vi "Dashboard Main.vi"() -> ()   [LabVIEW 2014]
uses:
  <vilib>/Rock Robotics/WPI/DriverStation/WPI_DriverStationRobotMode2.ctl
  <vilib>/event_ctls.llb/eventvkey.ctl
  <vilib>/Rock Robotics/WPI/Dashboard/WPI_DashboardLogging Global.vi
  <vilib>/Rock Robotics/Network Tables/SD Write Number.vi
  <vilib>/Rock Robotics/Network Tables/NT Read Numeric Array.vi
  <vilib>/Rock Robotics/Network Tables/SD Read Number.vi
  <vilib>/Rock Robotics/Network Tables/SD Write Boolean.vi
  <vilib>/Utility/config.llb/Write Key (String).vi
  <vilib>/Utility/config.llb/Write Key (I32).vi
  <vilib>/Utility/config.llb/Read Key (I32).vi
  <vilib>/Utility/config.llb/Read Key (Double).vi
  <vilib>/Utility/config.llb/Write Key (Double).vi
  <vilib>/Utility/config.llb/NI_LVConfig.lvlib
panel:
  in  "TCP":refnum<k5>
  out "Camera IP":string
  out "Image Message":string="Timeout in Camera Communications"
  in  "Dashboard Tab":T1(tab)
  in  "Straight Forward":bool
  in  "Camera Settings":T2={"Frame Rate"=30, "Compression"=30, "Size"=1} {"Frame Rate" scale=1.0..30.0; "Size" items=["640x480", "320x240", "160x120"]}
  out "MotorChart R":cluster{"Numeric":dbl, "Numeric":dbl}(graph)
  out "MotorChart L":T3(graph)
  out "MotorSliders R":cluster{"MotorSlide1":dbl, "MotorSlide2":dbl} {"MotorSlide2" scale=-1.0..1.0 scale format="%#_2e"; "MotorSlide1" scale=-1.0..1.0 scale format="%#_2e"}
  out "MotorSliders L":T4 {"MotorSlide4 2" scale=0.0..14.0 scale format="%#_2e"; "MotorSlide2" scale=-1.0..1.0 scale format="%#_2e"; "MotorSlide1" scale=-1.0..1.0 scale format="%#_2e"}
  out "Yaw":dbl(knob) scale=180.0..-180.0
  out "JS1 Z":dbl(slide) scale=-1.0..1.0 scale format="%#_2e"
  out "JS1 Graph":cluster{"X":dbl, "Y":dbl}[](graph)
  out "JS1 Buttons":T5
  out "JS2 Z":dbl(slide) scale=-1.0..1.0 scale format="%#_2e"
  out "JS2 Graph":cluster{"X":dbl, "Y":dbl}[](graph)
  out "JS2 Buttons":T5
  out "Mode":T6(ring)=enum."Auto Disabled"
  in  "DB Camera Config":bool
  out "fps":dbl format="%#.1g"
  out "Mbps":dbl format="%#.1g"
  out "Mbps 2":bool
  in  "Use This Auto":enum16{"Grab", "Knock", "Drive", "Test"}(ring)
  in  "Load":bool
  in  "Save":bool
  in  "Actions":T7(array[ring])
  in  "Bin Z":dbl
  in  "Gap Y":dbl
  in  "Auto Zone Y":dbl
  in  "Bin 4 Coordinates":dbl[](array[numeric])=[117.35, 90.0]
  in  "Bin 3 Coordinates":dbl[](array[numeric])=[48.65, 90.0]
  in  "Bin 2 Coordinates":dbl[](array[numeric])=[-48.65, 90.0]
  in  "Bin 1 Coordinates":dbl[](array[numeric])=[-117.35, 90.0]
  in  "Middle 2 Bins":enum16{"Strafe By", "Go Into Gap"}(ring)
  in  "Auto Zone":enum16{"0", "1", "2", "3", "4"}(ring)
  in  "Start Position":T8(ring)
  in  "In. to go forward":dbl format="%#_13g"
  out "CAN Device Errors":dbl[](array[numeric])
  out "Waveform Chart":T9(graph)
  in  "Test Slider":dbl(slide) scale=0.0..100.0 scale format="%#_3g"
  in  "On/Off":bool caption="Solenoid"
  in  "Test Name":u16(ring) items=["Select the test to run...", "Example Test", "-------------------------------", "List of tests is built in robot code.", "Replace with your own automated tests."]
  in  "Test Tree":string(tree)
  in  "Motor":cluster{"Value":dbl, "Enable":bool} {"Value" scale=-1.0..1.0 scale format="%#_3g"}
  out "Progress":T10 {"Test Progress" scale=0.0..100.0}
  in  "Rev/Fwd":cluster{"Forward":bool, "Reverse":bool}
  in  "Test Ring":u16(ring) items=["Monochrome", "Color"]
  in  "Vision":u16(ring) items=["Camera Off", "USB Camera SW", "USB Camera HW", "IP Camera"]
  in  "Rec Mode":enum32{"Stop", "Record", "Playback"}(radio)
  in  "Listbox":i32(listbox)
  out "Tree":string(tree)
  out "Camera Image":T11(plugin-control)
  out "Boolean":bool
  # "Left"
  # "Front"
  # "Right"
  # "Battery"
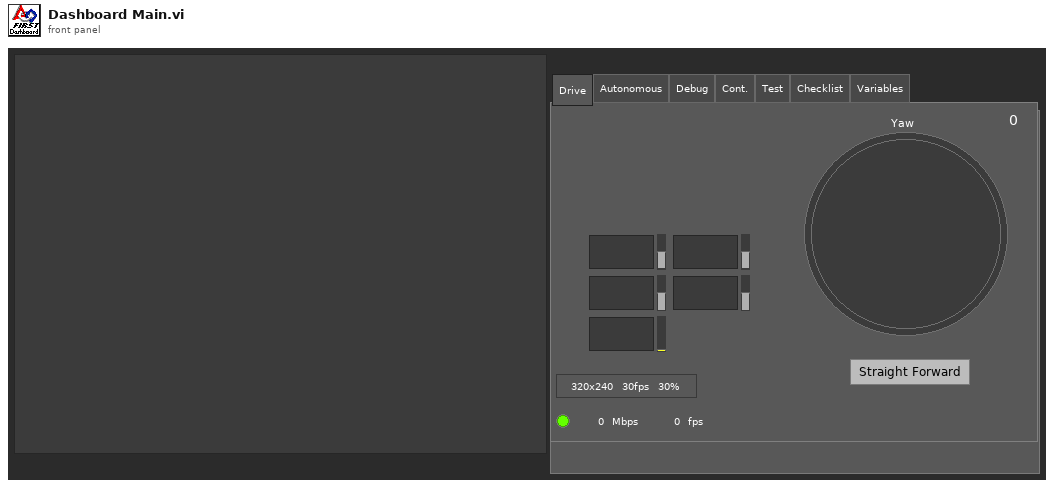
[diagram p1: front panel]
types:
  T1 = enum32{"Drive", "Autonomous", "Debug", "Cont.", "Test", "Checklist", "Variables"}
  T2 = cluster{"Frame Rate":i32, "Compression":i32, "Size":u16}
  T3 = cluster{"Numeric":dbl, "Numeric":dbl, "Battery V":dbl}
  T4 = cluster{"MotorSlide1":dbl, "MotorSlide2":dbl, "MotorSlide4 2":dbl}
  T5 = cluster{bool, bool, bool, bool, bool, bool, bool, bool, bool, bool, bool, bool}
  T6 = enum8{"Tele-Op Disabled", "Tele-Op Enabled", "Auto Disabled", "Auto Enabled", "Test Disabled", "Test Enabled", "Disconnected", "No Code", "E-Stop"}
  T7 = enum16{"Go To Auto Zone", "Grab Bin 1", "Grab Bin 2", "Grab Bin 3", "Grab Bin 4"}[]
  T8 = enum16{"Bin 1", "Bin 2", "Middle", "Bin 3", "Bin 4"}
  T9 = cluster{"Numeric Array[0]":dbl, "Numeric Array[1]":dbl, "Numeric Array[2]":dbl, "Numeric Array[3]":dbl, "Numeric Array[4]":dbl, "Numeric Array[5]":dbl, "Numeric Array[6]":dbl, "Numeric Array[7]":dbl, "Numeric Array[8]":dbl, "Numeric Array[9]":dbl}
  T10 = cluster{"Test Progress":u8, "Test Progress Text":string}
  T11 = typedef "IMAQ Image.ctl" = refnum<image>
  T12 = enum32{"Drive", "Basic", "Custom", "Test", "Checklist", "Variables"}
  T13 = typedef "Image Type" = u32
  T14 = typedef "NI_LVConfig.lvlib/Config Data RefNum.ctl" = refnum<k1>
  T15 = typedef "WPI_DriverStationRobotMode2.ctl" = enum16{"Autonomous Disabled", "Autonomous Enabled", "Teleop Disabled", "Teleop Enabled", "Disconnected", "Finish", "Test Disabled", "Test Enabled", "Emergency Stopped"}
  T16 = enum16{"Go To Auto Zone", "Grab Bin 1", "Grab Bin 2", "Grab Bin 3", "Grab Bin 4"}
  T17 = cluster{"Camera Image":refnum<vi>, "Dashboard Tab":refnum<vi>, "Boolean":refnum<vi>, "Vision":refnum<vi>, "Rec Mode":refnum<vi>, "Test Slider":refnum<vi>, "On/Off ":refnum<vi>, "Test Ring":refnum<vi>, "Rev/Fwd":refnum<vi>, "Test Name":refnum<vi>, "Motor":refnum<vi>, "Progress":refnum<vi>, "CheckList":refnum<vi>, "Tree":refnum<vi>, "Test Tree":refnum<vi>}
  T18 = cluster{"Error Strings":string, "Disable Counts":cluster{u16, u16}, "Rail Faults":cluster{u16, u16, u16}, "Robot IP":string, "DB Mode":u8, "Event Info":cluster{"Name":string, "Type":u8, "Number":u16, "Replay":u8}, "Camera Addr":string}
  T19 = cluster{"Storage":cluster{"Disk Free":u64, "RAM Block":u32, "RAM free":u32}, "CPU Utilization":cluster{"CPU % ISR":sgl, "CPU % Time Crit":sgl, "CPU % Timed Str":sgl, "CPU % High":sgl, "CPU % Above":sgl, "CPU % Normal":sgl, "CPU % Low":sgl}, "CAN":cluster{"% Bus Utilization":sgl, "Bus Off Cnt":u32, "TX_FIFO Full Cnt":u32, "Receive Error Cnt":u8, "Transmit Error Cnt":u8}, "HID":cluster{"HID Outputs":u32, "Rumble Low":u16, "Rumble High":u16}[]}
  T20 = cluster{"Status bits":cluster{"Test Mode":bool, "Autonomous":bool, "Enabled":bool, "Code Start":bool, "Brownout":bool, "Reserved 2":bool, "Reserved 3":bool, "E-Stop":bool}, "Code Trace":cluster{"Disabled":bool, "TeleOp":bool, "Auto":bool, "Test":bool}, "Controller Type":enum16{"unknown", "cRIO", "roboRio"}, "Code?":enum16{"unknown", "noCode", "code"}, "Battery V":dbl}
  T21 = cluster{"Control Bits":cluster{"TestMode":bool, "Autonomous":bool, "Enabled":bool, "FMS Present":bool, bool, bool, bool, "E-Stop":bool}, "Team Station ":u8, "Countdown":sgl, "Joystick Values":cluster{"Axes":dbl[], "Buttons":bool[], "POVs":i16[]}[]}
  T22 = cluster{"Axes":dbl[], "Buttons":bool[], "POVs":i16[]}[]
  T23 = cluster{"Axes":dbl[], "Buttons":bool[], "POVs":i16[]}
  T24 = cluster{"Buttons[0]":bool, "Buttons[1]":bool, "Buttons[2]":bool, "Buttons[3]":bool, "Buttons[4]":bool, "Buttons[5]":bool, "Buttons[6]":bool, "Buttons[7]":bool, "Buttons[8]":bool, "Buttons[9]":bool, "Buttons[10]":bool, "Buttons[11]":bool}
  T25 = cluster{"Operation":enum16{"Update", "Clear"}, "Color Box":u32}[]
  T26 = typedef "eventvkey.ctl" = enum16{"ASCII", "Enter", "Return", "Shift", "Ctrl", "Alt", "Cmd", "Opt", "Caps", "NumLock", "Clear", "Break", "Up", "Down", "Left", "Right", "Insert", "Delete", "Home", "End", "PageUp", "PageDown", "Escape", "Help", "Pause", "ScrollLock", "F1", "F2", "F3", "F4", "F5", "F6", "F7", "F8", "F9", "F10", "F11", "F12", "F13", "F14", "F15", "F16", "F17", "F18", "F19", "F20", "F21", "F22", "F23", "F24", "Play", "VolumeUp", "VolumeDown", "Mute", "Two Byte Char"}
  T27 = cluster{"Image Size":bool, "Image Type":bool, "Pixel Value":bool, "ROI Information":bool, "Zoom Factor":bool}
  T28 = enum8{"Enabled", "Disabled", "Disabled and Grayed Out"}
  T29 = cluster{"Operation":enum16{"Update", "Clear"}, "Color Box":u32}
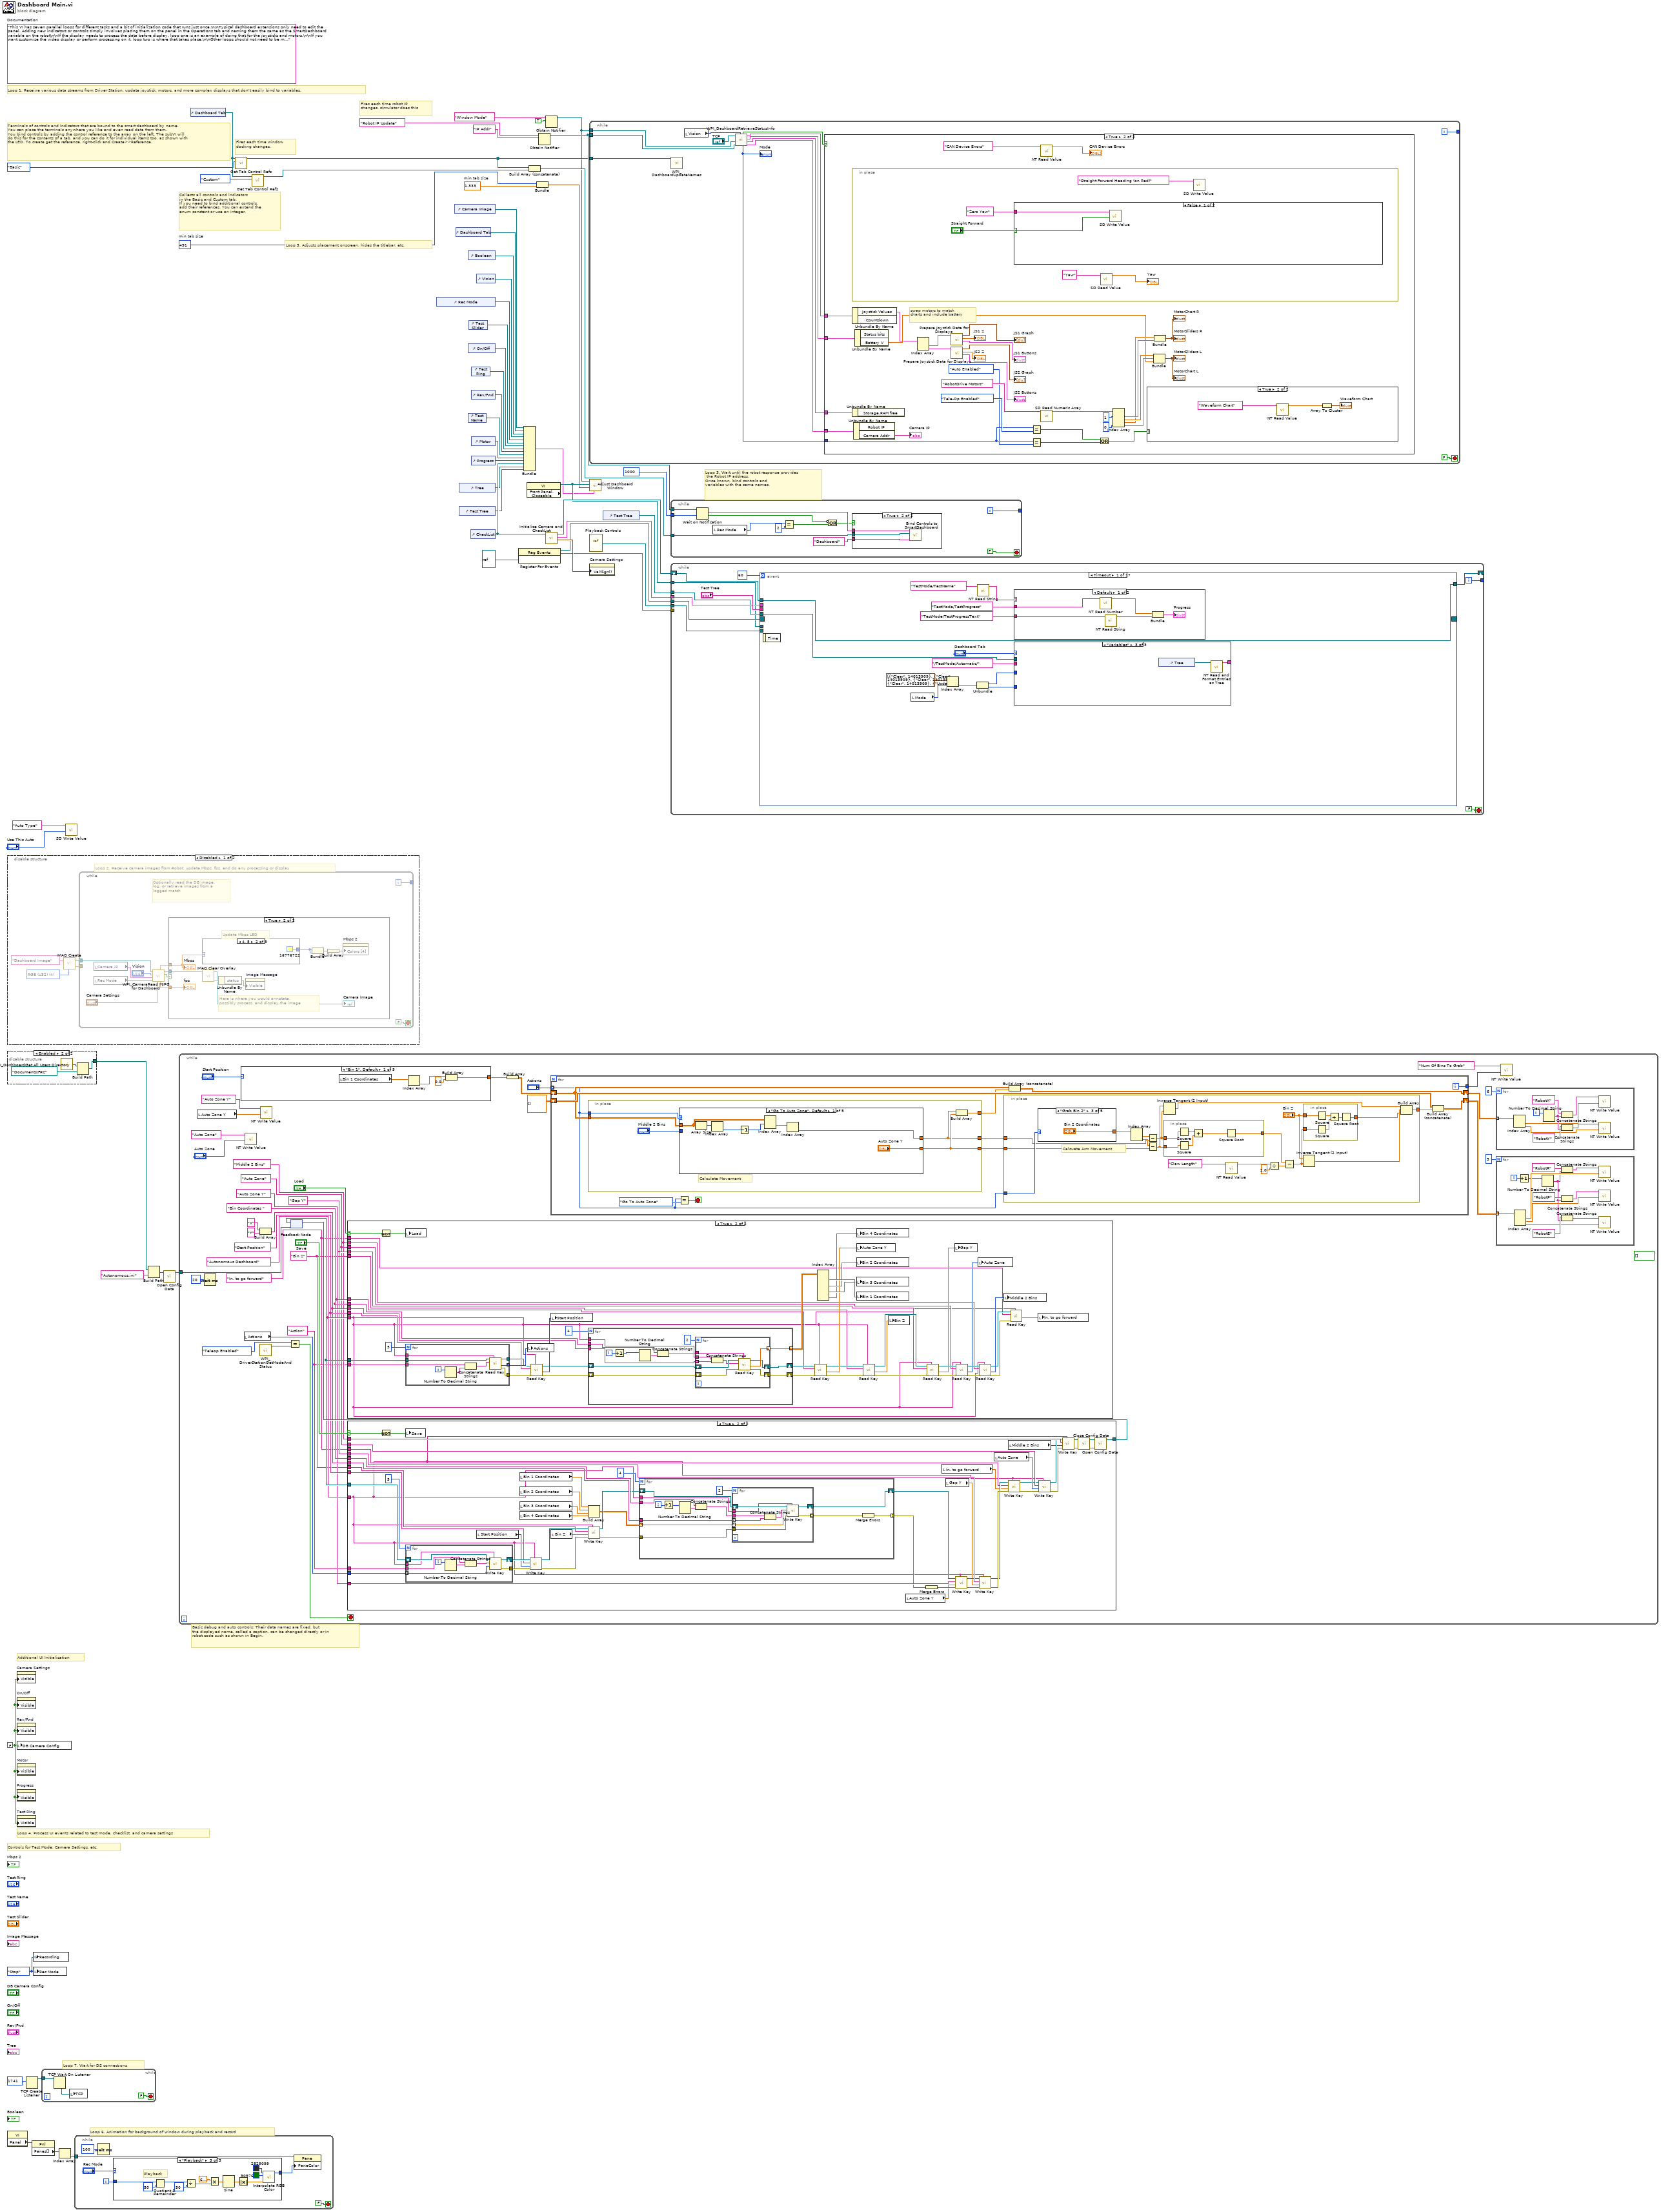
[diagram p0: block diagram]
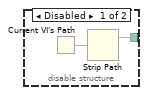
[diagram p2: hidden frame]
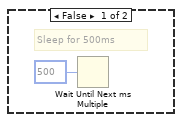
[diagram p3: hidden frame]
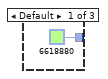
[diagram p4: hidden frame]
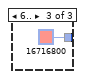
[diagram p5: hidden frame]
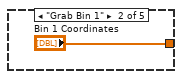
[diagram p10: hidden frame]
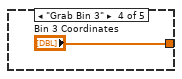
[diagram p11: hidden frame]
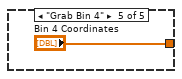
[diagram p12: hidden frame]
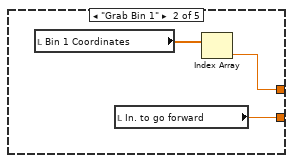
[diagram p13: hidden frame]
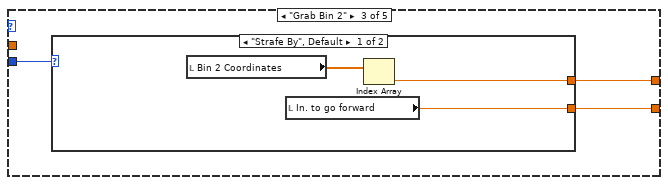
[diagram p14: hidden frame]
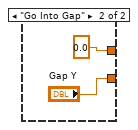
[diagram p15: hidden frame]
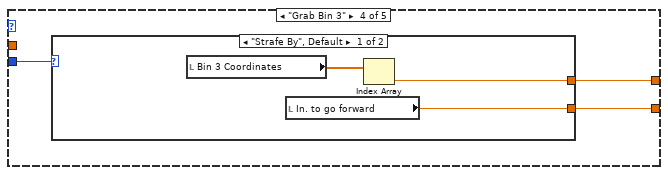
[diagram p16: hidden frame]
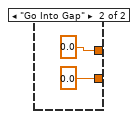
[diagram p17: hidden frame]
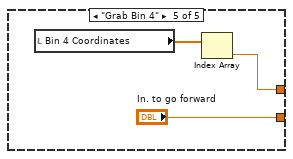
[diagram p18: hidden frame]
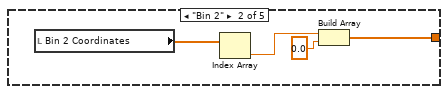
[diagram p19: hidden frame]
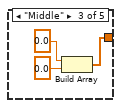
[diagram p20: hidden frame]
diagram:
  w30 = 491  # min tab size
  w29 = 1.333  # min tab size
  w38 = enum32{"Stop", "Record", "Playback"}."Stop" ("Rec Mode")
  w12 = FALSE ("Visible")
  (unwired) "This VI has seven parallel loops for different tasks and a bit of initialization code that runs just once.\n\nTypical dashboard extensions only need to edit the panel. Adding new indicators or controls simply involves placing them on the panel in the Operations tab and naming them the same as the SmartDashboard variable on the robot\n\nIf the display needs to process the data before display, loop one is an example of doing that for the joysticks and motors.\n\nIf you want customize the video display or perform processing on it, loop two is where that takes place.\n\nOther loops should not need to be modified. They are pretty standard, and document the task they perform."  # Documentation
  # "Loop 7. Wait for DS connections"
  # "Basic debug and auto controls: Their data names are fixed, but\nthe displayed name, called a caption, can be changed directly or in\nrobot code such as shown in Begin."
  # "Controls for Test Mode, Camera Settings, etc."
  # "Additional UI Initialization"
  # "Loop 6. Animation for background of window during playback and record"
  # "Fires each time robot IP\nchanges, simulator does this"
  # "Fires each time window\ndocking changes."
  # "Collects all controls and indicators\nin the Basic and Custom tab.\nIf you need to bind additional controls,\nadd their references. You can extend the\nenum constant or use an integer."
  # "Loop 4. Process UI events related to test mode, checklist, and camera settings"
  # "Terminals of controls and indicators that are bound to the smart dashboard by name.\nYou can place the terminals anywhere you like and even read data from them.\nYou bind controls by adding the control reference to the array on the left. The subVI will\ndo this for the contents of a tab, and you can do it for individual items too, as shown with\nthe LED. To create get the reference, right-click and Create>>Reference."
  # "Loop 3. Wait until the robot response provides\n the Robot IP address.\nOnce known, bind controls and\nvariables with the same names."
  # "Loop 5. Adjusts placement onscreen, hides the titlebar, etc."
  # "Loop 1. Receive various data streams from Driver Station, update joystick, motors, and more complex displays that don't easily bind to variables."
  n1 = disable-structure shown="Disabled" {
    frame Disabled {
      w58 = T13 4 items=["Grayscale (U8)", "Grayscale (I16)", "Grayscale (SGL)", "Complex (CSG)", "RGB (U32)", "HSL (U32)", "RGB (U64)"] ("Image Type")
      # "Loop 2. Receive camera images from Robot, update Mbps, fps, and do any processing or display"
      n2 = call "IMAQ Create"("Image Name"="Dashboard Image", "Image Type"=w58) -> ("New Image"=w56:T11, "error out"=w55:errorcluster)  [unwired: 2 in, 1 out]
      n3 = while {
        tunnel: w56 -> [w67]
        tunnel: w55 -> [_]
        tunnel: [w68] -> _
        i -> [w68]
        stop <- FALSE stop-if-true
        # "Optionally read the DB image,\nlog, or retrieve images from a\nlogged match"
        n4 = local read "Camera IP"() -> (w59:string)
        n5 = local read "Rec Mode"() -> (w61:enum32{"Stop", "Record", "Playback"})
        n6 = call <vilib>:"WPI_CameraRead MJPG for Dashboard.vi"("Camera Settings"="Camera Settings", "Rec Mode"=w61, "Camera IP"=w59, "Camera Mode"="Vision", "Refnum in"=w67) -> ("Active"=w65:bool, "Refnum out"=w66:T11, "FPS"=w64:dbl, "Bandwidth (Mbps)"=w63:dbl)  [unwired: 3 in]
        n7 = case shown="True" w65 {
          tunnel: w66 -> [_ w74]
          tunnel: w63 -> [_ w73]
          tunnel: w64 -> [_ w71]
          frame False {
            # "Sleep for 500ms"
            n8 = Wait Until Next ms Multiple(millisecond multiple=u32 500) -> ()  [unwired: 1 out]
          }
          frame True {
            # "Here is where you would annotate,\npossibly process, and display the image"
            # "Update Mbps LED"
            n9 = case shown="4, 5" w73 {
              tunnel: [u32 6618880 ("Color Box") u32 16776722 ("Color Box") u32 16716800 ("Color Box")] -> w75
              frame Default {
              }
              frame 4, 5 {
              }
              frame 6.. {
              }
            }
            n10 = call "IMAQ Clear Overlay"("Image"=w74) -> ("error out"=w78:errorcluster, "Image Out"=→"Camera Image":T11)  [unwired: 2 in, 7 out]
            n11 = Unbundle By Name(w78) -> ("status"=w79:bool)
            n12 = property on="Image Message" class="Str"("Visible"=w79) -> ()  [unwired: 2 in, 2 out]
            n13 = Bundle("Color Box"=w75, "Color Box"=w75) -> (w77:cluster{"Color Box":u32, "Color Box":u32})  [unwired: 1 out]
            n14 = Build Array(w77) -> (w76:cluster{"Color Box":u32, "Color Box":u32}[])
            n15 = property on="Mbps 2" class="Bool (strict)"("Colors [4]"=w76) -> ()  [unwired: 2 in, 2 out]
            "Mbps" <- w73
            "fps" <- w71
          }
        }
      }
    }
    frame Enabled {
    }
  }
  n16 = disable-structure shown="Enabled" {
    disable-tunnel: [w84 w87] -> w3
    frame Disabled {
      n17 = Current VI's Path() -> (path=w83:path)
      n18 = Strip Path(path=w83) -> (stripped path=w84:path)  [unwired: 1 out]
    }
    frame Enabled {
      n19 = call <vilib>:"WPI_DashboardGet All Users Directory.vi"() -> ("All User Path"=w85:path)
      n20 = Build Path(base path=w85, name or relative path=path "Documents/FRC" ("path")) -> (appended path=w87:path)
    }
  }
  n21 = property class="VI"() -> ("Panel"=w45:refnum<vi>)  [unwired: 2 in, 2 out]
  n22 = property on="Camera Settings" class="Clust (strict)"("Visible"=w12) -> ()  [unwired: 2 in, 2 out]
  n23 = property on="On/Off" class="Bool (strict)"("Visible"=w12) -> ()  [unwired: 2 in, 2 out]
  n24 = property on="Rev/Fwd" class="Clust (strict)"("Visible"=w12) -> ()  [unwired: 2 in, 2 out]
  n25 = local write "DB Camera Config"(w12) -> ()
  n26 = property on="Motor" class="Clust (strict)"("Visible"=w12) -> ()  [unwired: 2 in, 2 out]
  n27 = property on="Progress" class="Clust (strict)"("Visible"=w12) -> ()  [unwired: 2 in, 2 out]
  n28 = property on="Test Ring" class="Ring (strict)"("Visible"=w12) -> ()  [unwired: 2 in, 2 out]
  n29 = TCP Create Listener(10:u16 1741 ("timeout ms (25000)")) -> (3:w7:refnum<k5>)  [unwired: 4 in, 2 out]
  n30 = property class="Pnl"(reference=w45) -> ("Panes[]"=w46:refnum<vi>[])  [unwired: 1 in, 2 out]
  n31 = global write "WPI_DashboardLogging Global.vi" "Recording"(w38) -> ()
  n32 = local write "Rec Mode"(w38) -> ()
  n33 = while {
    tunnel: w7 -> [w89]
    stop <- FALSE stop-if-true
    n34 = TCP Wait On Listener(11:w89) -> (4:w88:refnum<k5>)  [unwired: 3 in, 4 out]
    n35 = local write "TCP"(w88) -> ()
  }
  n36 = Index Array(array=w46) -> (element=w44:refnum<vi>)  [unwired: 1 in]
  n37 = call-poly <vilib>:"SD Write Value.vi"("Numeric"="Use This Auto", "Name"="Auto Type") -> ()  [unwired: 8 in, 2 out]
  n38 = while {
    tunnel: w44 -> [w92]
    i -> [w95]
    stop <- FALSE stop-if-true
    n39 = Wait (ms)(milliseconds to wait=u32 100) -> ()  [unwired: 1 out]
    n40 = case shown="\"Playback\"" "Rec Mode" {
      tunnel: w95 -> [_ _ w110]
      tunnel: [u32 2829099 ("Base Color") u32 11141120 ("Target Color") w99] -> w91
      frame "Stop", Default {
        # "Reset the color, extra updates don't cost much"
      }
      frame "Record" {
      }
      frame "Playback" {
        # "Playback"
        n41 = Quotient & Remainder(x=w110, y=u32 50 ("milliseconds to wait")) -> (x-y*floor(x/y)=w106:u32)  [unwired: 1 out]
        n42 = Divide(x=w106, y=u32 50 ("milliseconds to wait")) -> (x/y=w103:dbl)
        n43 = Multiply(x=6.283185307179586, y=w103) -> (x*y=w108:dbl)
        n44 = Sine(x=w108) -> (sin(x)=w107:dbl)
        n45 = Absolute Value(x=w107) -> (abs(x)=w100:dbl)
        n46 = call "Interpolate RGB Color.vi"("Proportion"=w100, "Target Color"=u32 30976, "Base Color"=u32 2829099) -> ("Result Color"=w99:u32)  [unwired: 8 in]
      }
    }
    n47 = property class="Pane"(reference=w92, "PaneColor"=w91) -> ()  [unwired: 1 in, 2 out]
  }
  n48 = Build Path(base path=w3, name or relative path="Autonomous.ini") -> (appended path=w6:path)
  n49 = call <vilib>:"Open Config Data.vi"("configuration file path"=w6) -> ("refnum"=w4:T14)  [unwired: 8 in, 2 out]
  n50 = while {
    tunnel: w4 -> [w131]
    stop <- w146 stop-if-true
    w115 = "In. to go forward" ("key")
    w117 = "Middle 2 Bins" ("key")
    w118 = "Auto Zone" ("key")
    w119 = "Gap Y" ("key")
    w121 = "Auto Zone Y" ("key")
    w122 = "Bin Coordinates " ("key")
    w120 = "Bin Z" ("key")
    w126 = "Start Position"
    w127 = "Autonomous Dashboard" ("section")
    w116 = "Action" ("string")
    (unwired) bool[] [] ("Boolean Array")
    n51 = local read "Auto Zone Y"() -> (w113:dbl)
    n52 = Wait (ms)(milliseconds to wait=u32 20) -> ()  [unwired: 1 out]
    n53 = case shown="\"Bin 1\", Default" "Start Position" {
      tunnel: [w415 w419 w422 w426 w431] -> w135
      frame "Bin 1", Default {
        n54 = local read "Bin 1 Coordinates"() -> (w414:dbl[])
        n55 = Index Array(array=w414) -> (element=w413:dbl)  [unwired: 1 in]
        n56 = Build Array(w413, 0.0 ("element")) -> (w415:dbl[])
      }
      frame "Bin 2" {
        n57 = local read "Bin 2 Coordinates"() -> (w418:dbl[])
        n58 = Index Array(array=w418) -> (element=w417:dbl)  [unwired: 1 in]
        n59 = Build Array(w417, 0.0 ("element")) -> (w419:dbl[])
      }
      frame "Middle" {
        n60 = Build Array(0.0 ("element"), 0.0 ("element")) -> (w422:dbl[])
      }
      frame "Bin 3" {
        n61 = local read "Bin 3 Coordinates"() -> (w425:dbl[])
        n62 = Index Array(array=w425) -> (element=w424:dbl)  [unwired: 1 in]
        n63 = Build Array(w424, 0.0 ("element")) -> (w426:dbl[])
      }
      frame "Bin 4" {
        n64 = local read "Bin 4 Coordinates"() -> (w429:dbl[])
        n65 = Index Array(array=w429) -> (element=w428:dbl)  [unwired: 1 in]
        n66 = Build Array(w428, 0.0 ("element")) -> (w431:dbl[])
      }
    }
    n67 = local read "Actions"() -> (w140:T7)
    n68 = call-poly <vilib>:"NT Write Value.vi"("Numeric"="Auto Zone", "Name"="Auto Zone") -> ()  [unwired: 9 in, 1 out]
    n69 = Build Array("X" ("key"), "Y" ("key")) -> (w123:string[])
    n70 = call <vilib>:"WPI_DriverStationGetModeAndStatus.vi"() -> ("Robot Mode"=w148:T15)  [unwired: 10 in, 1 out]
    n71 = call-poly <vilib>:"NT Write Value.vi"("Numeric"=w113, "Name"="Auto Zone Y") -> ()  [unwired: 9 in, 1 out]
    n72 = Equal?(x=WPI_DriverStationRobotMode2."Teleop Enabled", y=w148) -> (x = y?=w146:bool)
    n73 = feedback #1(w131) -> (w129:T14)
    n74 = case shown="True" "Load" {
      selector: "Load" -> [_ w211]
      tunnel: w129 -> [_ w215]
      tunnel: w127 -> [_ w171]
      tunnel: w126 -> [_ w208]
      tunnel: w122 -> [_ w203]
      tunnel: w123 -> [_ w202]
      tunnel: w121 -> [_ w194]
      tunnel: w120 -> [_ w189]
      tunnel: w119 -> [_ w185]
      tunnel: w118 -> [_ w182]
      tunnel: w117 -> [_ w178]
      tunnel: w116 -> [_ w176]
      tunnel: w115 -> [_ w173]
      frame False {
      }
      frame True {
        n75 = Not(x=w211) -> (.not. x?=w212:bool)
        n76 = local write "Load"(w212) -> ()
        n77 = for {
          N: 5 -> [_]
          tunnel: w215 -> [w246]
          tunnel: [w245] -> w213 mode=indexing
          tunnel: w171 -> [w243]
          tunnel: w176 -> [w241]
          tunnel: [w239] -> w210
          tunnel: [w238] -> w209
          i -> [w244]
          n78 = Number To Decimal String(number=w244) -> (decimal integer string=w240:string)  [unwired: 1 in]
          n79 = Concatenate Strings(w241, w240) -> (w242:string)
          n80 = call-poly <vilib>:"Read Key.vi"("section"=w243, "key"=w242, "refnum"=w246) -> ("error out"=w238:errorcluster, "value"=w245:i32, "refnum out"=w239:T14)  [unwired: 5 in, 1 out]
        }
        n81 = local write "Actions"(w213) -> ()
        n82 = call-poly <vilib>:"Read Key.vi"("section"=w171, "error in (no error)"=w209, "key"=w208, "refnum"=w210) -> ("error out"=w205:errorcluster, "value"=w207:i32, "refnum out"=w206:T14)  [unwired: 4 in, 1 out]
        n83 = local write "Start Position"(w207) -> ()
        n84 = for {
          N: 4 -> [_]
          tunnel: w203 -> [w225]
          tunnel: w171 -> [w224]
          tunnel: w202 -> [w219]
          tunnel: [w218] -> w201 mode=indexing
          shift-right: [w217] -> w196
          shift-left: w206 -> [w228]
          shift-right: [w216] -> w195
          shift-left: w205 -> [w227]
          i -> [w221]
          n85 = Increment(x=w221) -> (x+1=w222:i32)
          n86 = Number To Decimal String(number=w222) -> (decimal integer string=w220:string)  [unwired: 1 in]
          n87 = Concatenate Strings(w225, w220) -> (w223:string)
          n88 = for {
            N: 2 -> [_]
            tunnel: w223 -> [w235]
            tunnel: w224 -> [w234]
            tunnel: w219 -> [w232] mode=indexing
            tunnel: [w231] -> w218 mode=indexing
            shift-right: [w230] -> w217
            shift-left: w228 -> [w237]
            shift-right: [w229] -> w216
            shift-left: w227 -> [w236]
            n89 = Concatenate Strings(w235, w232) -> (w233:string)
            n90 = call-poly <vilib>:"Read Key.vi"("section"=w234, "error in (no error)"=w236, "key"=w233, "refnum"=w237) -> ("error out"=w229:errorcluster, "value"=w231:dbl, "refnum out"=w230:T14)  [unwired: 4 in, 1 out]
          }
        }
        n91 = call-poly <vilib>:"Read Key.vi"("section"=w171, "error in (no error)"=w195, "key"=w194, "refnum"=w196) -> ("error out"=w191:errorcluster, "value"=w193:dbl, "refnum out"=w192:T14)  [unwired: 4 in, 1 out]
        n92 = Index Array(array=w201) -> (element #1=w200:dbl[], element #2=w199:dbl[], element #3=w198:dbl[], element #4=w197:dbl[])  [unwired: 8 in]
        n93 = local write "Bin 4 Coordinates"(w197) -> ()
        n94 = local write "Auto Zone Y"(w193) -> ()
        n95 = local write "Bin 2 Coordinates"(w199) -> ()
        n96 = local write "Bin 3 Coordinates"(w198) -> ()
        n97 = local write "Bin 1 Coordinates"(w200) -> ()
        n98 = call-poly <vilib>:"Read Key.vi"("section"=w171, "error in (no error)"=w191, "key"=w189, "refnum"=w192) -> ("error out"=w187:errorcluster, "value"=w190:dbl, "refnum out"=w188:T14)  [unwired: 4 in, 1 out]
        n99 = local write "Bin Z"(w190) -> ()
        n100 = call-poly <vilib>:"Read Key.vi"("section"=w171, "error in (no error)"=w187, "key"=w185, "refnum"=w188) -> ("error out"=w183:errorcluster, "value"=w186:dbl, "refnum out"=w184:T14)  [unwired: 4 in, 1 out]
        n101 = local write "Gap Y"(w186) -> ()
        n102 = call-poly <vilib>:"Read Key.vi"("section"=w171, "error in (no error)"=w183, "key"=w182, "refnum"=w184) -> ("error out"=w179:errorcluster, "value"=w181:i32, "refnum out"=w180:T14)  [unwired: 4 in, 1 out]
        n103 = local write "Auto Zone"(w181) -> ()
        n104 = call-poly <vilib>:"Read Key.vi"("section"=w171, "error in (no error)"=w179, "key"=w178, "refnum"=w180) -> ("error out"=w175:errorcluster, "value"=w177:i32, "refnum out"=w174:T14)  [unwired: 4 in, 1 out]
        n105 = local write "Middle 2 Bins"(w177) -> ()
        n106 = call-poly <vilib>:"Read Key.vi"("section"=w171, "error in (no error)"=w175, "key"=w173, "refnum"=w174) -> ("value"=w172:dbl)  [unwired: 4 in, 3 out]
        n107 = local write "In. to go forward"(w172) -> ()
      }
    }
    n108 = case shown="True" "Save" {
      selector: "Save" -> [_ w291]
      tunnel: w129 -> [w247 w298]
      tunnel: w140 -> [_ w297]
      tunnel: [w247 w293] -> w130
      tunnel: w127 -> [_ w248]
      tunnel: w116 -> [_ w290]
      tunnel: w126 -> [_ w287]
      tunnel: w120 -> [_ w286]
      tunnel: w123 -> [_ w285]
      tunnel: w122 -> [_ w284]
      tunnel: w121 -> [_ w283]
      tunnel: w119 -> [_ w282]
      tunnel: w118 -> [_ w281]
      tunnel: w117 -> [_ w280]
      tunnel: w115 -> [_ w249]
      frame False {
      }
      frame True {
        n109 = Not(x=w291) -> (.not. x?=w292:bool)
        n110 = local write "Save"(w292) -> ()
        n111 = for {
          N: 5 -> [_]
          tunnel: w297 -> [w329] mode=indexing
          tunnel: [w327] -> w288
          tunnel: w248 -> [w325]
          tunnel: w290 -> [w323]
          shift-right: [w326] -> w289
          shift-left: w298 -> [w330]
          i -> [w328]
          n112 = Number To Decimal String(number=w328) -> (decimal integer string=w322:string)  [unwired: 1 in]
          n113 = Concatenate Strings(w323, w322) -> (w324:string)
          n114 = call-poly <vilib>:"Write Key.vi"("section"=w325, "value"=w329, "key"=w324, "refnum"=w330) -> ("error out"=w327:errorcluster, "refnum out"=w326:T14)  [unwired: 5 in, 1 out]
        }
        n115 = local read "Start Position"() -> (w279:T8)
        n116 = local read "Bin 1 Coordinates"() -> (w272:dbl[])
        n117 = local read "Bin 2 Coordinates"() -> (w271:dbl[])
        n118 = local read "Bin 3 Coordinates"() -> (w270:dbl[])
        n119 = local read "Bin 4 Coordinates"() -> (w269:dbl[])
        n120 = call-poly <vilib>:"Write Key.vi"("section"=w248, "error in (no error)"=w288, "value"=w279, "key"=w287, "refnum"=w289) -> ("error out"=w277:errorcluster, "refnum out"=w278:T14)  [unwired: 4 in, 1 out]
        n121 = local read "Bin Z"() -> (w276:dbl)
        n122 = Build Array(w272, w271, w270, w269) -> (w268:dbl[][])
        n123 = call-poly <vilib>:"Write Key.vi"("section"=w248, "error in (no error)"=w277, "value"=w276, "key"=w286, "refnum"=w278) -> ("error out"=w273:errorcluster, "refnum out"=w274:T14)  [unwired: 4 in, 1 out]
        n124 = for {
          N: 4 -> [_]
          tunnel: w273 -> [w311]
          tunnel: w284 -> [w309]
          tunnel: w248 -> [w308]
          tunnel: w285 -> [w303]
          tunnel: [w300] -> w267 mode=indexing
          tunnel: w268 -> [w301] mode=indexing
          shift-right: [w299] -> w265
          shift-left: w274 -> [w312]
          i -> [w305]
          n125 = Increment(x=w305) -> (x+1=w306:i32)
          n126 = Number To Decimal String(number=w306) -> (decimal integer string=w304:string)  [unwired: 1 in]
          n127 = Concatenate Strings(w309, w304) -> (w307:string)
          n128 = for {
            N: 2 -> [_]
            tunnel: w311 -> [w320]
            tunnel: w307 -> [w319]
            tunnel: w308 -> [w318]
            tunnel: w303 -> [w316] mode=indexing
            tunnel: [w315] -> w302 mode=indexing
            tunnel: w301 -> [w314] mode=indexing
            shift-right: [w313] -> w299
            shift-left: w312 -> [w321]
            n129 = Concatenate Strings(w319, w316) -> (w317:string)
            n130 = call-poly <vilib>:"Write Key.vi"("section"=w318, "error in (no error)"=w320, "value"=w314, "key"=w317, "refnum"=w321) -> ("error out"=w315:errorcluster, "refnum out"=w313:T14)  [unwired: 4 in, 1 out]
          }
          n131 = Merge Errors(w302) -> (w300:errorcluster)
        }
        n132 = local read "Auto Zone Y"() -> (w264:dbl)
        n133 = Merge Errors(w267) -> (w266:errorcluster)
        n134 = local read "In. to go forward"() -> (w250:dbl)
        n135 = local read "Gap Y"() -> (w261:dbl)
        n136 = call-poly <vilib>:"Write Key.vi"("section"=w248, "error in (no error)"=w266, "value"=w264, "key"=w283, "refnum"=w265) -> ("error out"=w262:errorcluster, "refnum out"=w263:T14)  [unwired: 4 in, 1 out]
        n137 = call-poly <vilib>:"Write Key.vi"("section"=w248, "error in (no error)"=w262, "value"=w261, "key"=w282, "refnum"=w263) -> ("error out"=w254:errorcluster, "refnum out"=w253:T14)  [unwired: 4 in, 1 out]
        n138 = local read "Auto Zone"() -> (w260:enum16{"0", "1", "2", "3", "4"})
        n139 = local read "Middle 2 Bins"() -> (w257:enum16{"Strafe By", "Go Into Gap"})
        n140 = call-poly <vilib>:"Write Key.vi"("section"=w248, "error in (no error)"=w254, "value"=w250, "key"=w249, "refnum"=w253) -> ("error out"=w251:errorcluster, "refnum out"=w252:T14)  [unwired: 4 in, 1 out]
        n141 = call-poly <vilib>:"Write Key.vi"("section"=w248, "error in (no error)"=w251, "value"=w260, "key"=w281, "refnum"=w252) -> ("error out"=w259:errorcluster, "refnum out"=w258:T14)  [unwired: 4 in, 1 out]
        n142 = call-poly <vilib>:"Write Key.vi"("section"=w248, "error in (no error)"=w259, "value"=w257, "key"=w280, "refnum"=w258) -> ("error out"=w255:errorcluster, "refnum out"=w256:T14)  [unwired: 4 in, 1 out]
        n143 = call <vilib>:"Close Config Data.vi"("error in (no error)"=w255, "refnum"=w256) -> ("error out"=w295:errorcluster, "file path"=w294:path)  [unwired: 8 in]
        n144 = call <vilib>:"Open Config Data.vi"("error in (no error)"=w295, "configuration file path"=w294) -> ("refnum"=w293:T14)  [unwired: 7 in, 2 out]
      }
    }
    n145 = feedback-in #1(w130) -> ()
    n146 = Build Array(w135) -> (w134:dbl[][])
    n147 = for {
      tunnel: "Actions" -> [w333] mode=indexing
      shift-right: [w337] -> w133
      shift-left: w134 -> [w335]
      shift-right: [w334] -> w132
      shift-left: dbl[][] [] -> [w338]
      tunnel: [w332] -> w112
      i -> [w332]
      stop <- w331 stop-if-true
      n148 = in-place {
        in-place-border: w335 -> [w379]
        in-place-border: w333 -> [w382]
        in-place-border: [w381] -> w342
        in-place-border: [w380] -> w341
        in-place-border: [w378] -> w336
        # "Calculate Movement"
        n149 = case shown="\"Go To Auto Zone\", Default" w382 {
          tunnel: [w385 w393 w394 w402 w412] -> w380
          tunnel: ["Auto Zone Y" w391 w395 w403 "In. to go forward"] -> w381
          tunnel: "Middle 2 Bins" -> [_ _ w396 w404 _]
          tunnel: w379 -> [w389 _ _ _ _]
          frame "Go To Auto Zone", Default {
            n150 = Array Size(array=w389) -> (size(s)=w388:i32[])
            n151 = Index Array(array=w388) -> (element=w387:i32)  [unwired: 1 in]
            n152 = Decrement(x=w387) -> (x-1=w384:i32)
            n153 = Index Array(array=w389, index (row)=w384) -> (element=w386:dbl[])  [unwired: 1 in]
            n154 = Index Array(array=w386) -> (element=w385:dbl)  [unwired: 1 in]
          }
          frame "Grab Bin 1" {
            n155 = local read "Bin 1 Coordinates"() -> (w392:dbl[])
            n156 = local read "In. to go forward"() -> (w391:dbl)
            n157 = Index Array(array=w392) -> (element=w393:dbl)  [unwired: 1 in]
          }
          frame "Grab Bin 2" {
            n158 = case shown="\"Strafe By\", Default" w396 {
              tunnel: [w397 "Gap Y"] -> w395
              tunnel: [w399 0.0] -> w394
              frame "Strafe By", Default {
                n159 = local read "Bin 2 Coordinates"() -> (w398:dbl[])
                n160 = local read "In. to go forward"() -> (w397:dbl)
                n161 = Index Array(array=w398) -> (element=w399:dbl)  [unwired: 1 in]
              }
              frame "Go Into Gap" {
              }
            }
          }
          frame "Grab Bin 3" {
            n162 = case shown="\"Strafe By\", Default" w404 {
              tunnel: [w405 0.0] -> w403
              tunnel: [w407 0.0 ("Numeric")] -> w402
              frame "Strafe By", Default {
                n163 = local read "Bin 3 Coordinates"() -> (w406:dbl[])
                n164 = local read "In. to go forward"() -> (w405:dbl)
                n165 = Index Array(array=w406) -> (element=w407:dbl)  [unwired: 1 in]
              }
              frame "Go Into Gap" {
              }
            }
          }
          frame "Grab Bin 4" {
            n166 = local read "Bin 4 Coordinates"() -> (w410:dbl[])
            n167 = Index Array(array=w410) -> (element=w412:dbl)  [unwired: 1 in]
          }
        }
        n168 = Build Array(w380, w381) -> (w378:dbl[])
      }
      n169 = Equal?(x=w333, y=T16."Go To Auto Zone") -> (x = y?=w331:bool)
      n170 = in-place {
        in-place-border: w333 -> [w360]
        in-place-border: w342 -> [w359]
        in-place-border: w341 -> [w358]
        in-place-border: [w343] -> w339
        # "Calcuate Arm Movement"
        n171 = case shown="\"Grab Bin 2\"" w360 {
          tunnel: [_ "Bin 1 Coordinates" "Bin 2 Coordinates" "Bin 3 Coordinates" "Bin 4 Coordinates"] -> w357
          frame "Go To Auto Zone", Default {
          }
          frame "Grab Bin 1" {
          }
          frame "Grab Bin 2" {
          }
          frame "Grab Bin 3" {
          }
          frame "Grab Bin 4" {
          }
        }
        n172 = Index Array(array=w357) -> (element #1=w356:dbl, element #2=w355:dbl)  [unwired: 2 in]
        n173 = Subtract(x=w356, y=w358) -> (x-y=w344:dbl)
        n174 = Subtract(x=w355, y=w359) -> (x-y=w345:dbl)
        n175 = Inverse Tangent (2 Input)(1:w344, 2:w345) -> (0:w361:dbl)
        n176 = in-place {
          in-place-border: [w374] -> w351
          in-place-border: w344 -> [w373]
          in-place-border: w345 -> [w372]
          n177 = Square(x=w373) -> (x^2=w377:dbl)
          n178 = Square(x=w372) -> (x^2=w376:dbl)
          n179 = Add(x=w377, y=w376) -> (x+y=w375:dbl)
          n180 = Square Root(x=w375) -> (sqrt(x)=w374:dbl)
        }
        n181 = call-poly <vilib>:"NT Read Value.vi"("Name"="Claw Length") -> ("Numeric"=w347:dbl)  [unwired: 9 in, 1 out]
        n182 = Divide(x=w347, y=2.0) -> (x/y=w349:dbl)
        n183 = Subtract(x=w351, y=w349) -> (x-y=w350:dbl)
        n184 = in-place {
          in-place-border: [w368] -> w352
          in-place-border: "Bin Z" -> [w367]
          in-place-border: w350 -> [w366]
          n185 = Square(x=w367) -> (x^2=w371:dbl)
          n186 = Square(x=w366) -> (x^2=w370:dbl)
          n187 = Add(x=w371, y=w370) -> (x+y=w369:dbl)
          n188 = Square Root(x=w369) -> (sqrt(x)=w368:dbl)
        }
        n189 = Inverse Tangent (2 Input)(1:w350, 2:"Bin Z") -> (0:w354:dbl)
        n190 = Build Array(w361, w354, w352) -> (w343:dbl[])
      }
      n191 = Build Array (concatenate)(w335, w336) -> (w337:dbl[][])
      n192 = Build Array (concatenate)(w338, w339) -> (w334:dbl[][])
    }
    n193 = for {
      N: 6 -> [_]
      tunnel: w133 -> [w164] mode=indexing
      i -> [w168]
      n194 = Index Array(array=w164) -> (element #1=w163:dbl, element #2=w162:dbl)  [unwired: 2 in]
      n195 = Number To Decimal String(number=w168) -> (decimal integer string=w166:string)  [unwired: 1 in]
      n196 = Concatenate Strings("RobotX" ("string"), w166) -> (w170:string)
      n197 = Concatenate Strings("RobotY" ("string"), w166) -> (w167:string)
      n198 = call-poly <vilib>:"NT Write Value.vi"("Numeric"=w163, "Name"=w170) -> ()  [unwired: 9 in, 1 out]
      n199 = call-poly <vilib>:"NT Write Value.vi"("Numeric"=w162, "Name"=w167) -> ()  [unwired: 9 in, 1 out]
    }
    n200 = for {
      N: 5 -> [_]
      tunnel: w132 -> [w157] mode=indexing
      i -> [w149]
      n201 = Index Array(array=w157) -> (element #1=w156:dbl, element #2=w155:dbl, element #3=w153:dbl)  [unwired: 3 in]
      n202 = Increment(x=w149) -> (x+1=w150:i32)
      n203 = Number To Decimal String(number=w150) -> (decimal integer string=w152:string)  [unwired: 1 in]
      n204 = Concatenate Strings("RobotR" ("string"), w152) -> (w161:string)
      n205 = Concatenate Strings("RobotP" ("string"), w152) -> (w159:string)
      n206 = Concatenate Strings("RobotE" ("string"), w152) -> (w151:string)
      n207 = call-poly <vilib>:"NT Write Value.vi"("Numeric"=w156, "Name"=w161) -> ()  [unwired: 9 in, 1 out]
      n208 = call-poly <vilib>:"NT Write Value.vi"("Numeric"=w155, "Name"=w159) -> ()  [unwired: 9 in, 1 out]
      n209 = call-poly <vilib>:"NT Write Value.vi"("Numeric"=w153, "Name"=w151) -> ()  [unwired: 9 in, 1 out]
    }
    n210 = call-poly <vilib>:"NT Write Value.vi"("Numeric"=w112, "Name"="Num Of Bins To Grab") -> ()  [unwired: 9 in, 1 out]
  }
  n211 = control-ref of="Dashboard Tab"() -> (w36:refnum<vi>)
  n212 = call <vilib>:"Get Tab Control Refs.vi"("Page Index"=T12."Basic" ("Dashboard Tab"), "TabControl in"=w36) -> ("ControlsOnPage"=w10:refnum<vi>[])  [unwired: 9 in]
  n213 = call <vilib>:"Get Tab Control Refs.vi"("Page Index"=T12."Custom" ("Dashboard Tab"), "TabControl in"=w36) -> ("ControlsOnPage"=w35:refnum<vi>[])  [unwired: 9 in]
  n214 = control-ref of="Rec Mode"() -> (w18:refnum<vi>)
  n215 = control-ref of="Camera Image"() -> (w33:refnum<vi>)
  n216 = control-ref of="Dashboard Tab"() -> (w32:refnum<vi>)
  n217 = control-ref of="Tree"() -> (w22:refnum<vi>)
  n218 = control-ref of="Test Tree"() -> (w21:refnum<vi>)
  n219 = control-ref of="Boolean"() -> (w27:refnum<vi>)
  n220 = control-ref of="On/Off"() -> (w16:refnum<vi>)
  n221 = control-ref of="Test Name"() -> (w20:refnum<vi>)
  n222 = control-ref of="Test Slider"() -> (w17:refnum<vi>)
  n223 = control-ref of="CheckList"() -> (w23:refnum<vi>)
  n224 = control-ref of="Test Ring"() -> (w15:refnum<vi>)
  n225 = control-ref of="Rev/Fwd"() -> (w14:refnum<vi>)
  n226 = control-ref of="Motor"() -> (w19:refnum<vi>)
  n227 = control-ref of="Progress"() -> (w13:refnum<vi>)
  n228 = control-ref of="Vision"() -> (w31:refnum<vi>)
  n229 = register-events(refnum<vi> refnum) -> (reference out=w42:refnum<event-registration>, error out=w41:errorcluster)  [unwired: 2 in]
  n230 = Bundle("Camera Image"=w33, "Dashboard Tab"=w32, "Boolean"=w27, "Vision"=w31, "Rec Mode"=w18, "Test Slider"=w17, "On/Off"=w16, "Test Ring"=w15, "Rev/Fwd"=w14, "Test Name"=w20, "Motor"=w19, "Progress"=w13, "CheckList"=w23, "Tree"=w22, "Test Tree"=w21) -> (w24:T17)  [unwired: 1 in]
  n231 = property class="VI" props=["Front Panel.Closeable"]() -> (reference out=w37:refnum<vi>)  [unwired: 2 in, 2 out]
  n232 = Build Array (concatenate)(w10, w35) -> (w34:refnum<vi>[])
  n233 = Bundle("min tab size"=w30, "min tab size"=w29) -> (w28:cluster{"min tab size":i32, "min tab size":dbl})  [unwired: 1 in]
  n234 = Obtain Notifier(name (unnamed)="Robot IP Update", notification data type="IP Addr" ("name (unnamed)")) -> (notifier out=w11:refnum<notifier>)  [unwired: 2 in, 2 out]
  n235 = Obtain Notifier(name (unnamed)="Window Mode", notification data type=TRUE) -> (notifier out=w9:refnum<notifier>)  [unwired: 2 in, 2 out]
  n236 = call "Initialize Camera and CheckList.vi"("ListBox in"=w23) -> ("Cluster"=w49:cluster{"value":i32, "value":i32, "index":i32}, "Array"=w50:cluster{string[]}[], "File Refnum"=w48:T14)  [unwired: 8 in]
  n237 = while {
    tunnel: [w443] -> _
    tunnel: w11 -> [w437]
    tunnel: w10 -> [w436]
    tunnel: w9 -> [w432]
    i -> [w443]
    stop <- FALSE stop-if-true
    n238 = call <vilib>:"WPI_DashboardUpdateNames.vi"("Controls on Tab"=w436) -> ()  [unwired: 11 in]
    n239 = local read "Vision"() -> (w434:u16)
    n240 = call <vilib>:"WPI_DashboardRetrieveStatusInfo.vi"("Vision"=w434, "Binding Refnum"=w437, "Window Mode Notifier"=w432, "TCP Cnx"="TCP") -> ("Power and Errors"=w438:T18, "Robot Metrics"=w441:T19, "Status Info"=w442:T20, "Control Info"=w439:T21, "Robot Mode"=w435:T6, "Process?"=w440:bool)  [unwired: 2 in]
    "Mode" <- w435
    n241 = case shown="True" w440 {
      tunnel: w442 -> [_ w477]
      tunnel: w441 -> [_ w476]
      tunnel: w439 -> [_ w475]
      tunnel: w438 -> [_ w474]
      tunnel: w435 -> [_ w448]
      frame False {
      }
      frame True {
        # "swap motors to match\ncharts and include battery"
        n242 = in-place {
          n243 = case shown="False" "Straight Forward" {
            selector: "Straight Forward" -> [w486 w488]
            tunnel: "Zero Yaw" ("Name") -> [w487 w489]
            frame False {
              n244 = call-poly <vilib>:"SD Write Value.vi"("Boolean"=w486, "Name"=w487) -> ()  [unwired: 8 in, 2 out]
            }
            frame True {
              n245 = flat-sequence {
                tunnel: w489 -> [w491]
                tunnel: w488 -> [w490]
                frame #0 {
                  n246 = call-poly <vilib>:"SD Write Value.vi"("Boolean"=w490, "Name"=w491) -> ()  [unwired: 8 in, 2 out]
                }
                frame #1 {
                  n247 = Wait (ms)(milliseconds to wait=u32 100) -> ()  [unwired: 1 out]
                }
              }
            }
          }
          n248 = call-poly <vilib>:"SD Read Value.vi"("Name"="Yaw") -> ("Numeric"=→"Yaw":dbl)  [unwired: 8 in, 2 out]
          n249 = call-poly <vilib>:"SD Write Value.vi"("Name"="Straight Forward Heading (on Red)") -> ()  [unwired: 9 in, 2 out]
        }
        n250 = Unbundle By Name(w475) -> ("Joystick Values"=w462:T22)  [unwired: 1 out]
        n251 = Unbundle By Name(w476) -> ()  [unwired: 1 out]
        n252 = Unbundle By Name(w474) -> ("Camera Addr"=→"Camera IP":string)  [unwired: 1 out]
        n253 = Unbundle By Name(w477) -> ("Battery V"=w463:dbl)  [unwired: 1 out]
        n254 = Index Array(array=w462) -> (element #1=w461:T23, element #2=w456:T23)  [unwired: 2 in]
        n255 = call "Prepare Joystick Data for Displays.vi"("Joystick Values"=w461) -> ("Buttons"=→"JS1 Buttons":T24, "Z Axis"=→"JS1 Z":dbl, "Cartesian Data"=→"JS1 Graph":cluster{"X axis":dbl, "X axis":dbl}[])  [unwired: 8 in]
        n256 = call "Prepare Joystick Data for Displays.vi"("Joystick Values"=w456) -> ("Buttons"=→"JS2 Buttons":T24, "Z Axis"=→"JS2 Z":dbl, "Cartesian Data"=→"JS2 Graph":cluster{"X axis":dbl, "X axis":dbl}[])  [unwired: 8 in]
        n257 = Equal?(x=w448, y=T6."Tele-Op Enabled") -> (x = y?=w452:bool)
        n258 = Equal?(x=w448, y=T6."Auto Enabled") -> (x = y?=w449:bool)
        n259 = call-poly <vilib>:"NT Read Value.vi"("Name"="CAN Device Errors") -> ("Numeric Array"=→"CAN Device Errors":dbl[])  [unwired: 9 in, 1 out]
        n260 = call <vilib>:"SD Read Numeric Array.vi"("Name"="RobotDrive Motors") -> ("Numeric Array"=w465:dbl[])  [unwired: 8 in, 2 out]
        n261 = Or(x=w452, y=w449) -> (x .or. y?=w450:bool)
        n262 = Index Array(array=w465, index #1=1, index #4=0) -> (element #1=w469:dbl, element #2=w470:dbl, element #3=w468:dbl, element #4=w473:dbl)  [unwired: 2 in]
        n263 = case shown="True" w450 {
          frame False {
          }
          frame True {
            n264 = call-poly <vilib>:"NT Read Value.vi"("Name"="Waveform Chart") -> ("Numeric Array"=w479:dbl[])  [unwired: 9 in, 1 out]
            n265 = Array To Cluster(array=w479) -> (cluster=→"Waveform Chart":T9)
          }
        }
        n266 = Bundle("Numeric"=w470, "Numeric"=w473, "Battery V"=w463) -> (→"MotorChart L" →"MotorSliders L":T3)  [unwired: 1 in]
        n267 = Bundle("Numeric"=w468, "Numeric"=w469) -> (→"MotorChart R" →"MotorSliders R":cluster{"Numeric":dbl, "Numeric":dbl})  [unwired: 1 in]
      }
    }
  }
  n268 = call "Adjust Dashboard Window.vi"("Sizing Refnums"=w24, "Size Constraints"=w28, "VI"=w37, "Notifier in"=w9) -> ()  [unwired: 8 in]
  n269 = vi-ref "Playback Controls.vi"() -> (w43:refnum<vi>)
  n270 = property on="Camera Settings" class="Clust (strict)"("Val(Sgnl)"=w49) -> ()  [unwired: 2 in, 2 out]
  n271 = control-ref of="Test Tree"() -> (w47:refnum<vi>)
  n272 = while {
    tunnel: w34 -> [w504]
    tunnel: w11 -> [w502]
    tunnel: [w500] -> _
    tunnel: u32 1000 ("milliseconds to wait") -> [w499]
    i -> [w500]
    stop <- FALSE stop-if-true
    n273 = Wait on Notification(notifier=w502, timeout in ms (-1)=w499) -> (notification=w501:string, timed out?=w497:bool)  [unwired: 2 in, 2 out]
    n274 = local read "Rec Mode"() -> (w495:enum32{"Stop", "Record", "Playback"})
    n275 = Equal?(x=w495, y=u16 2 ("Rec Mode")) -> (x = y?=w496:bool)
    n276 = Compound Arithmetic op=OR(invert w497, w496) -> (w498:bool)
    n277 = case shown="True" w498 {
      tunnel: w504 -> [_ w507]
      tunnel: w501 -> [_ w506]
      tunnel: "Dashboard" -> [_ w505]
      frame False {
      }
      frame True {
        n278 = call <vilib>:"Bind Controls to SmartDashboard.vi"("Client Name"=w505, "Bound Control Refs"=w507, "Server IP Address"=w506) -> ()  [unwired: 9 in]
      }
    }
  }
  n279 = while {
    tunnel: w50 -> [w515]
    shift-right: [w514] -> _
    shift-left: w48 -> [w513]
    tunnel: [w512] -> _
    tunnel: w47 -> [w511]
    tunnel: w43 -> [w510]
    tunnel: w42 -> [w509]
    tunnel: w41 -> [_]
    tunnel: w37 -> [w508]
    i -> [w512]
    stop <- FALSE stop-if-true
    n280 = event shown="[0] Timeout" {
      selector: w509 -> [_ _ _ _ _ _ _ _ _ _ _ _ _ _ _ _ _]
      dyn-events: [_ _ _ _ _ _ _ _ _ _ _ _ _ w753 _ _ _] -> _
      timeout: u32 60 ("milliseconds to wait") -> [_ _ _ _ _ _ _ _ _ _ _ _ _ _ _ _ _]
      tunnel: w511 -> [w527 _ _ _ _ _ _ _ _ _ _ _ _ _ _ _ _]
      tunnel: "Test Tree" -> [_ _ _ _ _ _ _ _ w722 w730 w732 w736 w744 _ _ _ _]
      tunnel: w515 -> [_ w549 _ _ _ _ w686 w716 _ _ _ _ _ _ _ _ _]
      tunnel: [w523 w548 w647 w652 w660 w672 w685 w709 w721 w728 w731 w735 w743 w755 w769 w770 w780] -> w514
      tunnel: w513 -> [w523 w548 w647 w652 w660 w672 w684 w709 w721 w728 w731 w735 w743 w755 w769 w770 w780]
      tunnel: w510 -> [_ _ _ _ _ _ _ _ _ _ _ _ _ w756 _ w773 _]
      tunnel: w508 -> [_ _ _ _ _ _ _ _ _ _ _ _ _ w751 _ _ _]
      event Timeout {
        n281 = event-data() -> ()  [unwired: 1 in, 1 out]
        n282 = local read "Mode"() -> (w526:T6)
        n283 = Index Array(array=T25 [{"Operation"=enum."Clear", "Color Box"=14013909}, {"Operation"=enum."Clear", "Color Box"=14013909}, {"Operation"=enum."Clear", "Color Box"=14013909}, {"Operation"=enum."Clear", "Color Box"=14013909}, {"Operation"=enum."Update", "Color Box"=14013909}, {"Operation"=enum."Update", "Color Box"=16777215}, {"Operation"=enum."Clear", "Color Box"=14013909}, {"Operation"=enum."Clear", "Color Box"=14013909}, {"Operation"=enum."Clear", "Color Box"=14013909}], index=w526) -> (element=w521:T29)
        n284 = Unbundle(w521) -> ("Operation"=w520:enum16{"Update", "Clear"}, "Color Box"=w519:u32)
        n285 = call <vilib>:"NT Read String.vi"("Name"="TestMode/TestName") -> ("String"=w530:string)  [unwired: 9 in, 1 out]
        n286 = case shown="Default" w530 {
          tunnel: "TestMode/TestProgress" ("Name") -> [w542 _]
          tunnel: "TestMode/TestProgressText" ("Name") -> [w541 _]
          frame Default {
            n287 = call <vilib>:"NT Read Number.vi"("Name"=w542) -> ("Numeric"=w543:dbl)  [unwired: 9 in, 1 out]
            n288 = call <vilib>:"NT Read String.vi"("Name"=w541) -> ("String"=w544:string)  [unwired: 9 in, 1 out]
            n289 = Bundle("Numeric"=w543, "String"=w544) -> (→"Progress":cluster{"Numeric":dbl, "String":string})  [unwired: 1 in]
          }
          frame "" {
            n290 = local write "Test Name"(u16 0) -> ()
            n291 = property on="Progress" class="Clust (strict)"("Visible"=FALSE) -> ()  [unwired: 2 in, 2 out]
          }
        }
        n292 = case shown="\"Variables\"" "Dashboard Tab" {
          tunnel: w527 -> [_ w538 _]
          tunnel: "/TestMode/Automatic/" ("Name Pattern") -> [_ w537 _]
          tunnel: w520 -> [_ w536 _]
          tunnel: [_ _ w540] -> _
          tunnel: w519 -> [_ w532 _]
          frame "Cont.", Default {
          }
          frame "Test" {
            w535 = -2 ("Active Item:Row Number")
            n293 = call <vilib>:"NT Read and Format Entries as Tree.vi"("Operation"=w536, "Name Pattern"=w537, "Tree Refnum"=w538) -> ()  [unwired: 7 in, 2 out]
            n294 = property on="Test Tree" class="Tree (strict)"("Active Item Row Number"=w535, "ActiveColNum"=w535, "CellBG"=w532, "Active Item Row Number"=-1 ("Active Item:Row Number"), "CellBG"=u32 5789784 ("Color Box")) -> ()  [unwired: 2 in, 2 out]
          }
          frame "Variables" {
            n295 = control-ref of="Tree"() -> (w539:refnum<vi>)
            n296 = call <vilib>:"NT Read and Format Entries as Tree.vi"("Tree Refnum"=w539) -> ("Formatted Strings"=w540:cluster{"Name":string, "Value":string}[])  [unwired: 9 in, 1 out]
          }
        }
      }
      event "Test Tree": Value Change {
        # "Show appropriate\ncontrols"
        n297 = event-data() -> ("CtlRef"=w552:refnum<vi>, "NewVal"=w550:string)  [unwired: 1 in]
        n298 = property on="Progress" class="Clust (strict)"("Visible"=FALSE) -> ()  [unwired: 2 in, 2 out]
        n299 = call <vilib>:"WPI_UtilitiesGetTreeIOName.vi"("NewVal"=w550, "TreeControl in"=w552) -> ("I/O Name"=w553:string)  [unwired: 9 in]
        n300 = case shown="\"Camera\"" w553 {
          selector: w553 -> [_ w560 _ w578 w587 _]
          tunnel: w550 -> [_ _ w575 w577 _ w594]
          tunnel: w549 -> [_ _ _ _ _ w593]
          frame Default {
            w555 = FALSE ("Visible")
            w554 = FALSE ("Visible")
            n301 = property on="Motor" class="Clust (strict)"("Visible"=w554) -> ()  [unwired: 2 in, 2 out]
            n302 = property on="On/Off" class="Bool (strict)"("Visible"=w555) -> ()  [unwired: 2 in, 2 out]
            n303 = property on="Test Ring" class="Ring (strict)"("Visible"=w554) -> ()  [unwired: 2 in, 2 out]
            n304 = property on="Test Slider" class="Slide (strict)"("Visible"=w555) -> ()  [unwired: 2 in, 2 out]
            n305 = property on="Rev/Fwd" class="Clust (strict)"("Visible"=w555) -> ()  [unwired: 2 in, 2 out]
          }
          frame "Motor", "PWM" {
            w561 = FALSE ("Visible")
            n306 = case shown="\"Motor\", Default" w560 {
              tunnel: [1.0 ("Value") -1.0 ("Value")] -> w559
              tunnel: [255.0 ("Value") 1.0 ("Value")] -> w558
              tunnel: [128.0 ("Value") 0.0 ("Value")] -> w557
              tunnel: [64.0 ("Value") 0.5 ("Value")] -> w556
              frame "PWM" {
              }
              frame "Motor", Default {
              }
            }
            n307 = property on="On/Off" class="Bool (strict)"("Visible"=w561) -> ()  [unwired: 2 in, 2 out]
            n308 = property on="Motor" class="Clust (strict)"("Visible"=TRUE) -> ()  [unwired: 2 in, 2 out]
            n309 = property on="Test Slider" class="Slide (strict)"("Visible"=w561) -> ()  [unwired: 2 in, 2 out]
            n310 = property on="Test Ring" class="Ring (strict)"("Visible"=w561) -> ()  [unwired: 2 in, 2 out]
            n311 = property on="Rev/Fwd" class="Clust (strict)"("Visible"=w561) -> ()  [unwired: 2 in, 2 out]
            n312 = property on="Value" class="Slide (strict)"("Value"=w557, "Scale.Minimum"=w559, "Scale.Maximum"=w558, "Scale.Increment"=w556) -> ()  [unwired: 2 in, 2 out]
          }
          frame "Servo" {
            w573 = FALSE ("Visible")
            n313 = call <vilib>:"NT Read Number.vi"("Name"=w575) -> ("Numeric"=w574:dbl)  [unwired: 9 in, 1 out]
            n314 = property on="Motor" class="Clust (strict)"("Visible"=w573) -> ()  [unwired: 2 in, 2 out]
            n315 = property on="On/Off" class="Bool (strict)"("Visible"=w573) -> ()  [unwired: 2 in, 2 out]
            n316 = property on="Test Slider" class="Slide (strict)"("Visible"=TRUE, "Scale.Maximum"=170.0 ("Scale.Range:Maximum")) -> ()  [unwired: 2 in, 2 out]
            n317 = local write "Test Slider"(w574) -> ()
            n318 = property on="Test Ring" class="Ring (strict)"("Visible"=w573) -> ()  [unwired: 2 in, 2 out]
            n319 = property on="Rev/Fwd" class="Clust (strict)"("Visible"=w573) -> ()  [unwired: 2 in, 2 out]
          }
          frame "Relay", "Solenoid" {
            w576 = FALSE ("Visible")
            n320 = property on="Motor" class="Clust (strict)"("Visible"=w576) -> ()  [unwired: 2 in, 2 out]
            n321 = property on="Test Slider" class="Slide (strict)"("Visible"=w576) -> ()  [unwired: 2 in, 2 out]
            n322 = property on="Test Ring" class="Ring (strict)"("Visible"=w576) -> ()  [unwired: 2 in, 2 out]
            n323 = Search and Replace String(input string=w577, search string="/Value  **", replace string="/Direction") -> (result string=w583:string)  [unwired: 5 in, 3 out]
            n324 = call <vilib>:"NT Read String.vi"("Name"=w583) -> ("String"=w581:string)  [unwired: 9 in, 1 out]
            n325 = Equal?(x="Both directions", y=w581) -> (x = y?=w579:bool)
            n326 = property on="Rev/Fwd" class="Clust (strict)"("Visible"=w579) -> ()  [unwired: 2 in, 2 out]
            n327 = Not(x=w579) -> (.not. x?=w580:bool)
            n328 = property on="On/Off" class="Bool (strict)"("Visible"=w580, "Caption.Text"=w578) -> ()  [unwired: 2 in, 2 out]
          }
          frame "Compressor", "Digital Out" {
            w586 = FALSE ("Visible")
            # "Get direction and finish"
            n329 = property on="Motor" class="Clust (strict)"("Visible"=w586) -> ()  [unwired: 2 in, 2 out]
            n330 = property on="Rev/Fwd" class="Clust (strict)"("Visible"=FALSE) -> ()  [unwired: 2 in, 2 out]
            n331 = property on="Test Ring" class="Ring (strict)"("Visible"=w586) -> ()  [unwired: 2 in, 2 out]
            n332 = property on="Test Slider" class="Slide (strict)"("Visible"=w586) -> ()  [unwired: 2 in, 2 out]
            n333 = property on="On/Off" class="Bool (strict)"("Visible"=TRUE, "Caption.Text"=w587) -> ()  [unwired: 2 in, 2 out]
          }
          frame "Camera" {
            n334 = call <vilib>:"Get Last Path Segment.vi"("String in"=w594) -> ("String out"=w595:string)  [unwired: 10 in]
            n335 = property on="Motor" class="Clust (strict)"("Visible"=FALSE) -> ()  [unwired: 2 in, 2 out]
            n336 = case shown="\"White Balance  **\"" w595 {
              tunnel: w594 -> [w601 w610 w619 w628 w637 _ w643]
              tunnel: w593 -> [w599 w607 w616 w625 w634 _ _]
              frame "Size  **" {
                n337 = Index Array(array=w599) -> (element=w598:cluster{string[]})  [unwired: 1 in]
                n338 = call <vilib>:"NT Read String.vi"("Name"=w601) -> ("String"=w600:string)  [unwired: 9 in, 1 out]
                n339 = property on="Test Ring" class="Ring (strict)"("Visible"=TRUE) -> ()  [unwired: 2 in, 2 out]
                n340 = property on="Test Slider" class="Slide (strict)"("Visible"=FALSE) -> ()  [unwired: 2 in, 2 out]
                n341 = Unbundle(w598) -> (w596:string[])
                n342 = Match First String(2:w596, 3:w600) -> (0:w597:i32)  [unwired: 1 out]
                n343 = property on="Test Ring" class="Ring (strict)"("Value"=w597, "Strings []"=w596) -> ()  [unwired: 2 in, 2 out]
              }
              frame "White Balance  **" {
                n344 = call <vilib>:"NT Read String.vi"("Name"=w610) -> ("String"=w609:string)  [unwired: 9 in, 1 out]
                n345 = Index Array(array=w607, index=1) -> (element=w608:cluster{string[]})
                n346 = property on="Test Ring" class="Ring (strict)"("Visible"=TRUE) -> ()  [unwired: 2 in, 2 out]
                n347 = property on="Test Slider" class="Slide (strict)"("Visible"=FALSE) -> ()  [unwired: 2 in, 2 out]
                n348 = Unbundle(w608) -> (w605:string[])
                n349 = Match First String(2:w605, 3:w609) -> (0:w604:i32)  [unwired: 1 out]
                n350 = property on="Test Ring" class="Ring (strict)"("Value"=w604, "Strings []"=w605) -> ()  [unwired: 2 in, 2 out]
              }
              frame "Exposure  **" {
                n351 = call <vilib>:"NT Read String.vi"("Name"=w619) -> ("String"=w618:string)  [unwired: 9 in, 1 out]
                n352 = Index Array(array=w616, index=2) -> (element=w617:cluster{string[]})
                n353 = property on="Test Ring" class="Ring (strict)"("Visible"=TRUE) -> ()  [unwired: 2 in, 2 out]
                n354 = property on="Test Slider" class="Slide (strict)"("Visible"=FALSE) -> ()  [unwired: 2 in, 2 out]
                n355 = Unbundle(w617) -> (w613:string[])
                n356 = Match First String(2:w613, 3:w618) -> (0:w614:i32)  [unwired: 1 out]
                n357 = property on="Test Ring" class="Ring (strict)"("Value"=w614, "Strings []"=w613) -> ()  [unwired: 2 in, 2 out]
              }
              frame "Exposure Priority  **" {
                n358 = call <vilib>:"NT Read String.vi"("Name"=w628) -> ("String"=w627:string)  [unwired: 9 in, 1 out]
                n359 = Index Array(array=w625, index=3) -> (element=w626:cluster{string[]})
                n360 = property on="Test Ring" class="Ring (strict)"("Visible"=TRUE) -> ()  [unwired: 2 in, 2 out]
                n361 = property on="Test Slider" class="Slide (strict)"("Visible"=FALSE) -> ()  [unwired: 2 in, 2 out]
                n362 = Unbundle(w626) -> (w622:string[])
                n363 = Match First String(2:w622, 3:w627) -> (0:w623:i32)  [unwired: 1 out]
                n364 = property on="Test Ring" class="Ring (strict)"("Value"=w623, "Strings []"=w622) -> ()  [unwired: 2 in, 2 out]
              }
              frame "Color Enable  **" {
                n365 = call <vilib>:"NT Read String.vi"("Name"=w637) -> ("String"=w636:string)  [unwired: 9 in, 1 out]
                n366 = Index Array(array=w634, index=4) -> (element=w635:cluster{string[]})
                n367 = property on="Test Ring" class="Ring (strict)"("Visible"=TRUE) -> ()  [unwired: 2 in, 2 out]
                n368 = property on="Test Slider" class="Slide (strict)"("Visible"=FALSE) -> ()  [unwired: 2 in, 2 out]
                n369 = Unbundle(w635) -> (w631:string[])
                n370 = Match First String(2:w631, 3:w636) -> (0:w632:i32)  [unwired: 1 out]
                n371 = property on="Test Ring" class="Ring (strict)"("Value"=w632, "Strings []"=w631) -> ()  [unwired: 2 in, 2 out]
              }
              frame Default {
                n372 = property on="Test Slider" class="Slide (strict)"("Visible"=FALSE) -> ()  [unwired: 2 in, 2 out]
                n373 = property on="Test Ring" class="Ring (strict)"("Visible"=FALSE) -> ()  [unwired: 2 in, 2 out]
              }
              frame "Brightness  **", "Color Level  **", "Compression  **", "FPS  **", "Sharpness  **" {
                n374 = call <vilib>:"NT Read Number.vi"("Name"=w643) -> ("Numeric"=w642:dbl)  [unwired: 9 in, 1 out]
                n375 = property on="Test Ring" class="Ring (strict)"("Visible"=FALSE) -> ()  [unwired: 2 in, 2 out]
                n376 = property on="Test Slider" class="Slide (strict)"("Visible"=TRUE, "Scale.Maximum"=100.0 ("Scale.Range:Maximum")) -> ()  [unwired: 2 in, 2 out]
                n377 = local write "Test Slider"(w642) -> ()
              }
            }
            n378 = property on="Rev/Fwd" class="Clust (strict)"("Visible"=FALSE) -> ()  [unwired: 2 in, 2 out]
            n379 = property on="On/Off" class="Bool (strict)"("Visible"=FALSE) -> ()  [unwired: 2 in, 2 out]
          }
        }
      }
      event "Test Name": Mouse Enter {
        # "Populate the ring with the list of tests"
        n380 = event-data() -> ()  [unwired: 1 in, 1 out]
        n381 = call <vilib>:"NT Read String Array.vi"("Name"="TestMode/TestList") -> ("String Array"=w651:string[])  [unwired: 9 in, 1 out]
        n382 = Build Array (concatenate)("Select the test to run...", w651) -> (w650:string[])
        n383 = property on="Test Name" class="Ring (strict)"("Strings []"=w650) -> ()  [unwired: 2 in, 2 out]
      }
      event "Test Name": Value Change {
        w653 = FALSE ("Visible")
        # "Tell the robot the test name to run"
        n384 = event-data() -> ("NewVal"=w657:u16)  [unwired: 1 in]
        n385 = property on="Progress" class="Clust (strict)"("Visible"=TRUE) -> ()  [unwired: 2 in, 2 out]
        n386 = local write "Progress"(T10 {"Test Progress"=0, "Test Progress Text"=""} ("Progress")) -> ()
        n387 = property on="Motor" class="Clust (strict)"("Visible"=w653) -> ()  [unwired: 2 in, 2 out]
        n388 = property on="On/Off" class="Bool (strict)"("Visible"=w653) -> ()  [unwired: 2 in, 2 out]
        n389 = property on="Test Name" class="Ring (strict)"() -> ("Strings []"=w658:string[])  [unwired: 2 in, 2 out]
        n390 = property on="Test Ring" class="Ring (strict)"("Visible"=w653) -> ()  [unwired: 2 in, 2 out]
        n391 = property on="Test Slider" class="Slide (strict)"("Visible"=w653) -> ()  [unwired: 2 in, 2 out]
        n392 = property on="Rev/Fwd" class="Clust (strict)"("Visible"=w653) -> ()  [unwired: 2 in, 2 out]
        n393 = Index Array(array=w658, index=w657) -> (element=w656:string)
        n394 = call <vilib>:"NT Write String.vi"("String"=w656, "Name"="TestMode/TestName") -> ()  [unwired: 9 in, 1 out]
      }
      event "Listbox": Double Click {
        # "Shift clears all"
        # "Update symbols on the listbox"
        n395 = event-data() -> ("PlatMods.Shift"=w661:bool, "Row"=w663:i32)  [unwired: 1 in]
        n396 = case shown="True" w661 {
          tunnel: w663 -> [w667 _]
          tunnel: 1 -> [w666 _]
          frame False {
            n397 = property on="Listbox" class="LstBox (strict)"() -> ("Item Symbols"=w665:i32[])  [unwired: 2 in, 2 out]
            n398 = Replace Array Subset(array=w665, new element=w666, index=w667) -> (w664:i32[])
            n399 = property on="Listbox" class="LstBox (strict)"("Item Symbols"=w664) -> ()  [unwired: 2 in, 2 out]
          }
          frame True {
            w668 = 0 ("Top Row")
            n400 = property on="Listbox" class="LstBox (strict)"() -> ("Number of Rows"=w670:u32)  [unwired: 2 in, 2 out]
            n401 = Initialize Array(0, w670) -> (w669:i32[])
            n402 = property on="Listbox" class="LstBox (strict)"("Top Row"=w668, "Value"=w668, "Item Symbols"=w669) -> ()  [unwired: 2 in, 2 out]
          }
        }
      }
      event "Listbox": Key Down {
        # "Update symbols on the listbox\nLeft and right keys check and uncheck"
        n403 = event-data() -> ("VKey"=w674:T26)  [unwired: 1 in]
        n404 = case shown="\"Left\", \"Right\"" w674 {
          selector: w674 -> [w679 _]
          tunnel: eventvkey."Left" ("VKey") -> [w677 _]
          frame "Left", "Right" {
            n405 = Equal?(x=w677, y=w679) -> (x = y?=w678:bool)
            n406 = Select(t=0, s=w678, f=1) -> (s? t:f=w680:i32)
            n407 = property on="Listbox" class="LstBox (strict)"() -> ("Item Symbols"=w683:i32[])  [unwired: 2 in, 2 out]
            n408 = Replace Array Subset(array=w683, new element=w680, index="Listbox") -> (w682:i32[])
            n409 = property on="Listbox" class="LstBox (strict)"("Item Symbols"=w682) -> ()  [unwired: 2 in, 2 out]
          }
          frame Default {
          }
        }
      }
      event "DB Camera Config": Value Change {
        # "Show or hide the cluster of controls, store in ini file"
        n410 = event-data() -> ("NewVal"=w687:bool)  [unwired: 1 in]
        n411 = case shown="False" w687 {
          tunnel: w686 -> [w696 _]
          tunnel: [w689 w707] -> w685
          tunnel: w684 -> [w688 w707]
          frame False {
            w703 = "Camera"
            w706 = FALSE ("Visible")
            n412 = property on="Camera Settings" class="Clust (strict)"("Visible"=w706) -> ()  [unwired: 2 in, 2 out]
            n413 = local write "DB Camera Config"(w706) -> ()
            n414 = local read "Camera Settings"() -> (w695:T2)
            n415 = Index Array(array=w696) -> (element=w699:cluster{string[]})  [unwired: 1 in]
            n416 = Unbundle(w699) -> (w698:string[])
            n417 = Unbundle(w695) -> ("Frame Rate"=w694:i32, "Compression"=w693:i32, "Size"=w697:u16)
            n418 = Index Array(array=w698, index=w697) -> (element=w692:string)
            n419 = call-poly <vilib>:"Write Key.vi"("section"=w703, "value"=w692, "key"="Size", "refnum"=w688) -> ("refnum out"=w705:T14)  [unwired: 2 in, 5 out]
            n420 = call-poly <vilib>:"Write Key.vi"("section"=w703, "value"=w694, "key"="FrameRate", "refnum"=w705) -> ("refnum out"=w704:T14)  [unwired: 1 in, 6 out]
            n421 = call-poly <vilib>:"Write Key.vi"("section"=w703, "value"=w693, "key"="Compression", "refnum"=w704) -> ("refnum out"=w690:T14)  [unwired: 1 in, 6 out]
            n422 = call <vilib>:"Close Config Data.vi"("refnum"=w690) -> ("file path"=w691:path)  [unwired: 2 in, 8 out]
            n423 = call <vilib>:"Open Config Data.vi"("configuration file path"=w691) -> ("refnum"=w689:T14)  [unwired: 8 in, 2 out]
          }
          frame True {
            n424 = property on="Camera Settings" class="Clust (strict)"("Visible"=TRUE) -> ()  [unwired: 2 in, 2 out]
          }
        }
      }
      event "Camera Settings": Value Change {
        # "Update summary string when any elements of DB camera change"
        n425 = event-data() -> ("NewVal"=w720:T2)  [unwired: 1 in]
        n426 = Index Array(array=w716) -> (element=w715:cluster{string[]})  [unwired: 1 in]
        n427 = Unbundle(w715) -> (w714:string[])
        n428 = Unbundle(w720) -> ("Frame Rate"=w711:i32, "Compression"=w710:i32, "Size"=w713:u16)
        n429 = Index Array(array=w714, index=w713) -> (element=w712:string)
        n430 = Format Into String(format string="%s   %dfps   %d%%", w712, w711, w710) -> (resulting string=w717:string)  [unwired: 2 in, 1 out]
        n431 = Build Array(w717) -> (w718:string[])
        n432 = property on="DB Camera Config" class="Bool (strict)"("Strings [4]"=w718) -> ()  [unwired: 2 in, 2 out]
      }
      event "Motor.Enable": Value Change {
        # "When the test mode otor enable helper is set, update that\ntree row item's value"
        n433 = event-data() -> ("NewVal"=w726:bool)  [unwired: 1 in]
        n434 = Unbundle("Motor") -> ("Value"=w725:dbl)  [unwired: 1 out]
        n435 = Select(t=w725, s=w726, f=0.0) -> (s? t:f=w723:dbl)
        n436 = call <vilib>:"NT Write Number.vi"("Numeric"=w723, "Name"=w722) -> ()  [unwired: 9 in, 1 out]
      }
      event "Test Slider": Value Change {
        # "When the test mode slider helper is set, update that\ntree row item's value"
        n437 = event-data() -> ("NewVal"=w729:dbl)  [unwired: 1 in]
        n438 = call <vilib>:"NT Write Number.vi"("Numeric"=w729, "Name"=w730) -> ()  [unwired: 9 in, 1 out]
      }
      event "On/Off": Value Change {
        # "When the test mode on/off helper value is set, update that\ntree row item's value"
        n439 = event-data() -> ("NewVal"=w734:bool)  [unwired: 1 in]
        n440 = Boolean To (0,1)(Boolean=w734) -> (0, 1=w733:i16)
        n441 = call <vilib>:"NT Write Number.vi"("Numeric"=w733, "Name"=w732) -> ()  [unwired: 9 in, 1 out]
      }
      event "Rev/Fwd": Value Change {
        # "When the test mode helper value for relays is set, update that\ntree row item's value"
        n442 = event-data() -> ("NewVal.Forward"=w742:bool, "NewVal.Reverse"=w741:bool)  [unwired: 1 in]
        n443 = Boolean To (0,1)(Boolean=w741) -> (0, 1=w740:i16)
        n444 = Boolean To (0,1)(Boolean=w742) -> (0, 1=w738:i16)
        n445 = Negate(x=w740) -> (-x=w739:i16)
        n446 = Add(x=w738, y=w739) -> (x+y=w737:i16)
        n447 = call <vilib>:"NT Write Number.vi"("Numeric"=w737, "Name"=w736) -> ()  [unwired: 9 in, 1 out]
      }
      event "Test Ring": Value Change {
        # "When a test mode helper value is selected from the ring,\nset the tree item's variable to the string value"
        n448 = event-data() -> ("NewVal"=w746:u16)  [unwired: 1 in]
        n449 = property on="Test Ring" class="Ring (strict)"() -> ("Strings []"=w747:string[])  [unwired: 2 in, 2 out]
        n450 = Index Array(array=w747, index=w746) -> (element=w745:string)
        n451 = call <vilib>:"NT Write String.vi"("String"=w745, "Name"=w744) -> ()  [unwired: 9 in, 1 out]
      }
      event "Rec Mode": Value Change {
        # "Update globals for recording mode and path to read log from.\nClear when logging and let NetworkTables set path for vision to\nuse."
        n452 = event-data() -> ("NewVal"=w757:enum32{"Stop", "Record", "Playback"})  [unwired: 1 in]
        n453 = global write "WPI_DashboardLogging Global.vi" "Logging Filename"(path "") -> ()
        n454 = global write "WPI_DashboardLogging Global.vi" "Recording"(w757) -> ()
        n455 = call <vilib>:"WPI_DashboardNT Log FieldName Cache.vi"("Operation"=enum16{"Lookup/Add", "Index", "Clear"}."Clear") -> ()  [unwired: 8 in, 3 out]
        n456 = case shown="\"Playback\"" w757 {
          tunnel: w756 -> [_ w759 w767]
          tunnel: [_ _ w766] -> w753
          tunnel: [_ _ w765] -> _
          tunnel: w751 -> [_ _ w763]
          tunnel: cluster{i32, i32} {-250, 170} -> [_ _ w762]
          tunnel: [_ _ T27 {"Image Size"=TRUE, "Image Type"=TRUE, "Pixel Value"=TRUE, "ROI Information"=TRUE, "Zoom Factor"=FALSE} ("Image Information Shown:All Elements")] -> w749
          tunnel: [_ _ TRUE ("Zoom Factor")] -> w748
          frame Default {
          }
          frame "Stop", "Record" {
            # "Place Window too"
            n457 = invoke class="VI" method="FP.Close"(reference=w759) -> (reference out=w758:refnum<vi>)  [unwired: 2 in, 2 out]
            n458 = invoke class="VI" method="Abort VI"(reference=w758) -> ()  [unwired: 2 in, 3 out]
          }
          frame "Playback" {
            n459 = call "Open Playback Panel.vi"("Offset"=w762, "DB VI Ref"=w763, "Playback in"=w767) -> ("Playback out"=w764:refnum<vi>)  [unwired: 8 in]
            n460 = register-events(w764) -> (reference out=w766:refnum<event-registration>, error out=w765:errorcluster)  [unwired: 2 in]
          }
        }
        n461 = property on="Camera Image" class="ImageControl"("Image Information Shown"=w749, "Image Information Visible"=w748) -> ()  [unwired: 2 in, 2 out]
      }
      event Panel Close {
        w768 = enum32{"Stop", "Record", "Playback"}."Stop" ("Rec Mode")
        # "Playback window has been closed, abort"
        n462 = event-data() -> ()  [unwired: 1 in, 4 out]
        n463 = local write "Rec Mode"(w768) -> ()
        n464 = global write "WPI_DashboardLogging Global.vi" "Recording"(w768) -> ()
      }
      event Panel Close {
        # "Abort playback window and ourself"
        n465 = event-data() -> ()  [unwired: 1 in, 4 out]
        n466 = invoke class="VI" method="FP.Close"(reference=w773) -> (reference out=w772:refnum<vi>)  [unwired: 2 in, 2 out]
        n467 = invoke class="VI" method="Abort VI"(reference=w772) -> (error out=w771:errorcluster)  [unwired: 2 in, 2 out]
        n468 = invoke class="VI" method="Abort VI"(error in=w771) -> ()  [unwired: 2 in, 3 out]
      }
      event "Vision": Value Change {
        # "Enable/Disable Compression slider.\nHW USB is hard-coded into the camera"
        n469 = event-data() -> ("NewVal"=w779:u16)  [unwired: 1 in]
        n470 = Equal?(x=w779, y=u32 2 ("milliseconds to wait")) -> (x = y?=w777:bool)
        n471 = Select(t=T28."Disabled and Grayed Out" ("Disabled"), s=w777, f=T28."Enabled" ("Disabled")) -> (s? t:f=w774:T28)
        n472 = property on="Compression" class="Slide (strict)"("DisabledEnum"=w774) -> ()  [unwired: 2 in, 2 out]
      }
    }
  }
